vi "Condicionais, While True.vi"() -> ()   [LabVIEW 2024]
panel:
  in  "Numeric 3":dbl
  in  "stop 2":bool
  out "Numeric 2":i32
  in  "milliseconds to wait 2":u32
  out "Celsius  2":dbl(slide) scale=-50.0..300.0 scale format="%#1.3g"
  in  "Fahrenheit 2":dbl(slide) scale=-50.0..500.0
  out "Celsius   2":dbl
  out "Fahrenheit  2":dbl
  in  "Boolean":bool
  out "Celsius":dbl
  out "Fahrenheit":dbl
  in  "Fahrenheit":dbl(slide) scale=-50.0..500.0
  out "Celsius":dbl(slide) scale=-50.0..300.0 scale format="%#1.3g"
  in  "milliseconds to wait":u32
  out "Numeric":i32
  in  "stop":bool
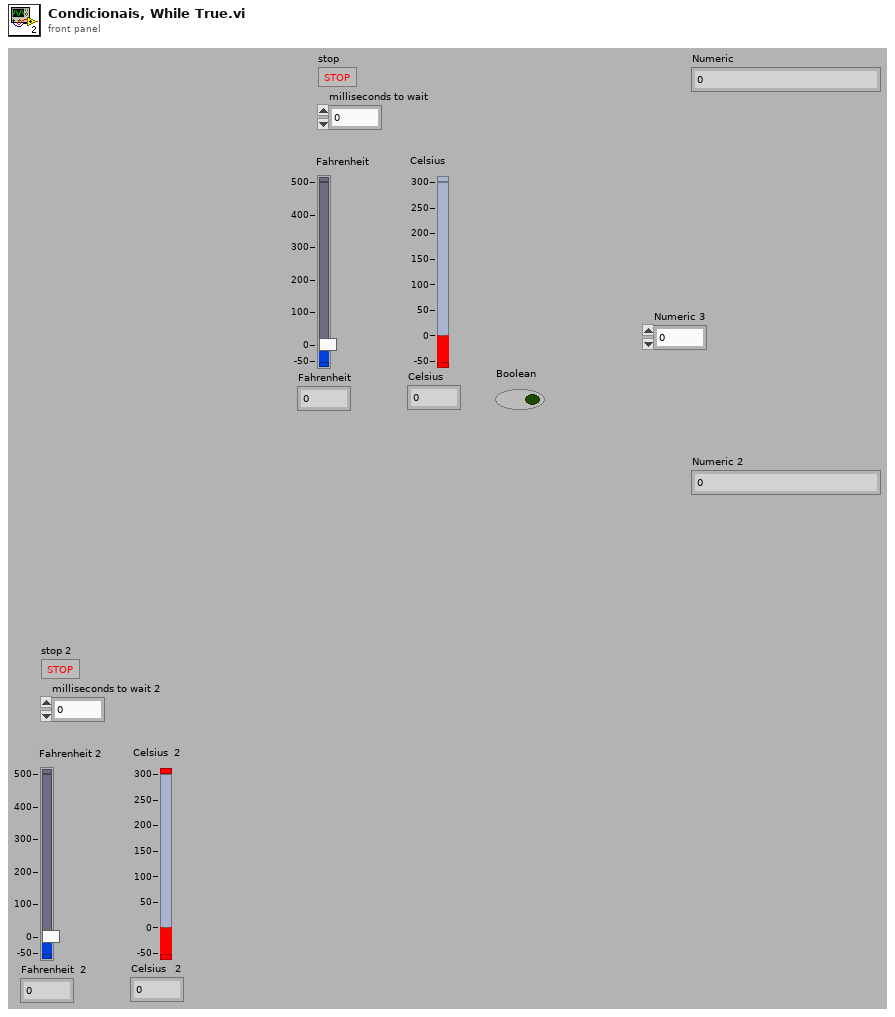
[diagram p1: front panel]
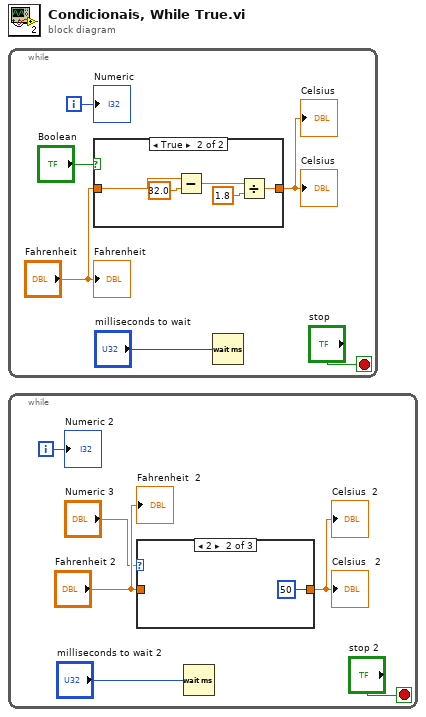
[diagram p0: block diagram]
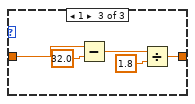
[diagram p3: hidden frame]
diagram:
  n1 = while {
    i -> [w5]
    stop <- "stop" stop-if-true
    n2 = case shown="True" "Boolean" {
      tunnel: [w7 w9] -> w3
      tunnel: "Fahrenheit" -> [w7 w8]
      frame False {
      }
      frame True {
        n3 = Subtract(x=w8, y=32.0) -> (x-y=w11:dbl)
        n4 = Divide(x=w11, y=1.8 ("x-y")) -> (x/y=w9:dbl)
      }
    }
    "Celsius" <- w3
    "Celsius" <- w3
    n5 = Wait (ms)(milliseconds to wait="milliseconds to wait") -> ()  [unwired: 1 out]
    "Numeric" <- w5
    "Fahrenheit" <- "Fahrenheit"
  }
  n6 = while {
    i -> [w17]
    stop <- "stop 2" stop-if-true
    n7 = case shown="2" "Numeric 3" {
      tunnel: [w19 50 w22] -> w15
      tunnel: "Fahrenheit 2" -> [w19 _ w21]
      frame 0, Default {
      }
      frame 2 {
      }
      frame 1 {
        n8 = Subtract(x=w21, y=32.0) -> (x-y=w24:dbl)
        n9 = Divide(x=w24, y=1.8 ("x-y")) -> (x/y=w22:dbl)
      }
    }
    "Celsius  2" <- w15
    "Celsius   2" <- w15
    n10 = Wait (ms)(milliseconds to wait="milliseconds to wait 2") -> ()  [unwired: 1 out]
    "Numeric 2" <- w17
    "Fahrenheit  2" <- "Fahrenheit 2"
  }
